vi "B_VI.vi"(9 "In B":i32, 10 "Internal B":refnum<vi>) -> ()   [LabVIEW 2015]
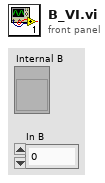
[diagram p1: front panel]
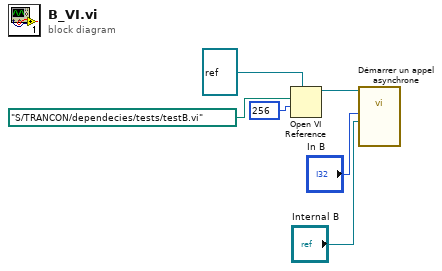
[diagram p0: block diagram]
diagram:
  n1 = Open VI Reference(type specifier VI Refnum (for type only)=refnum<vi> refnum ("spécificateur de type du refnum de VI (pour type seulement)"), vi path=path "S:/TRANCON/dependecies/tests/testB.vi" ("chemin du VI"), options=256) -> (vi reference=w2:refnum<vi>)  [unwired: 3 in, 1 out]
  n2 = call-by-ref "Démarrer un appel asynchrone"(reference=w2, "Internal 2"="Internal B", "Commande numérique 2"="In B") -> ()  [unwired: 10 in, 3 out]
